vi "Digital (Pipelined Sample Clock) - Continuous Output.vi"() -> ()   [LabVIEW 2022 SP3]
doc: "This example demonstrates how to interface the NI 6536/7 to a synchronous DAC with an output enabled signal."
uses:
  <vilib>/Utility/error.llb/DialogType.ctl
  <vilib>/DAQmx/write.llb/DAQmx Write (Digital 1D Wfm NChan NSamp).vi
  <vilib>/DAQmx/create/channels.llb/DAQmx Create Channel (DO-Digital Output).vi
  <vilib>/DAQmx/configure/timing.llb/DAQmx Timing (Pipelined Sample Clock).vi
  <vilib>/Waveform/DWDTOps.llb/Digital Pattern Generator (Ramp).vi
  <vilib>/Waveform/DWDTOps.llb/DWDT Uncompress Digital.vi
  <vilib>/DAQmx/miscellaneous.llb/DAQmx Fill In Error Info.vi
  <resource>/objmgr/daqmx.rc
panel:
  in  "Pause Trigger Polarity":i32(ring)=10192 items=["High"=10192, "Low"=10214]
  in  "Data Active Level":i32(ring)=10095 items=["Active High"=10095, "Active Low"=10096]
  in  "Sample Clock Polarity":i32(ring)=10095 items=["Active High"=10095, "Active Low"=10096]
  in  "Handshaking?":bool
  in  "Pause Trigger Source Terminal":tag="/Dev1/PFI1" caption="Pause Trigger \nSource"
  in  "Data Active Output Terminal":tag="/Dev1/PFI0" caption="Data Active Output"
  in  "Sample Clock Output":tag="/Dev1/PFI1"
  in  "Samples per Channel per write":u32=1000 caption="Samples per Buffer"
  in  "Stop":bool
  out "Digital Waveform Graph":digitalwaveform[](graph)
  in  "Sample Rate":dbl=1000.0
  in  "Line(s)":tag="Dev1/port0/line0:7"
  # "Channel Settings"
  # "Generated Data"
  # "Timing Settings"
  # "Advanced Settings"
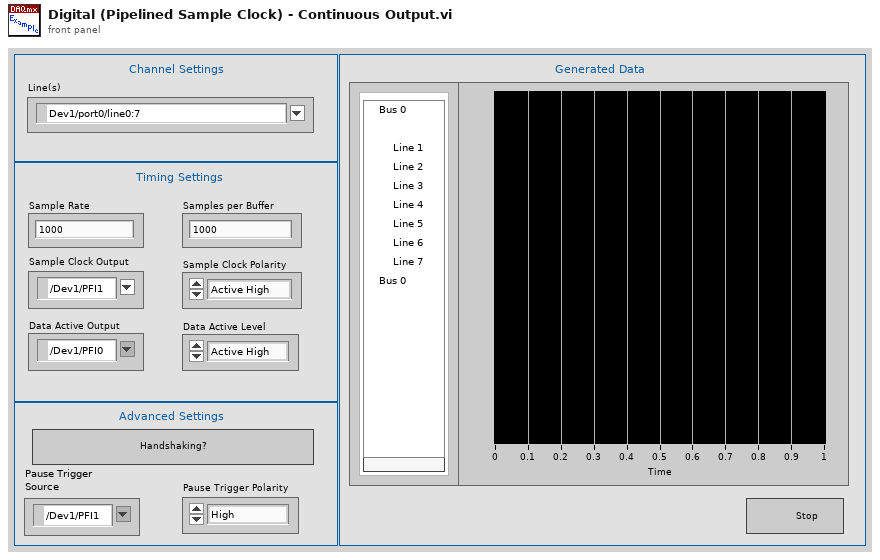
[diagram p1: front panel]
types:
  T1 = typedef "DialogType.ctl" = u16
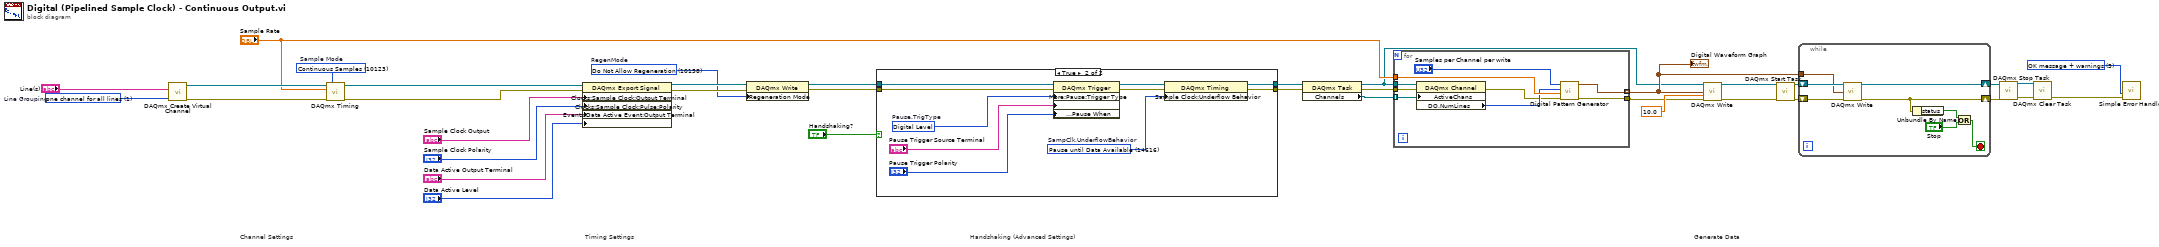
[diagram p0: block diagram]
diagram:
  w22 = T1 3 items=["no dialog", "OK message", "continue or stop message", "OK message + warnings", "continue/stop + warnings"] ("type of dialog (OK msg:1)")
  w10 = 10158 items=["Allow Regeneration"=10097, "Do Not Allow Regeneration"=10158]  # RegenMode
  w34 = 10123 items=["Finite Samples"=10178, "Continuous Samples"=10123, "Hardware Timed Single Point"=12522]  # Sample Mode
  w36 = 1 items=["one channel for each line", "one channel for all lines"]  # Line Grouping
  # "Timing Settings"
  # "Generate Data"
  # "Handshaking (Advanced Settings)"
  # "Channel Settings"
  n1 = call-poly <vilib>:"DAQmx Create Virtual Channel.vi"("lines"="Line(s)", "line grouping"=w36) -> ("task out"=w35:refnum<k21>, "error out"=w33:errorcluster)  [unwired: 12 in]
  n2 = call-poly <vilib>:"DAQmx Timing.vi"("task/channels in"=w35, "sample mode"=w34, "rate"="Sample Rate", "error in"=w33) -> ("task out"=w31:refnum<k21>, "error out"=w30:errorcluster)  [unwired: 10 in]
  n3 = property class="DAQmx Export Signal"(reference=w31, error in=w30, "Clocks:Sample Clock:Output Terminal"="Sample Clock Output", "Clocks:Sample Clock:Pulse:Polarity"="Sample Clock Polarity", "Events:Data Active Event:Output Terminal"="Data Active Output Terminal", "Events:Data Active Event:Level:Active Level"="Data Active Level") -> (reference out=w29:refnum<k21>, error out=w28:errorcluster)
  n4 = property class="DAQmx Write"(reference=w29, error in=w28, "Regeneration Mode"=w10) -> (reference out=w20:refnum<k21>, error out=w19:errorcluster)
  n5 = case shown="True" "Handshaking?" {
    tunnel: w20 -> [w38 w42]
    tunnel: w19 -> [w37 w45]
    tunnel: [w37 w43] -> w16
    tunnel: [w38 w40] -> w17
    frame False {
    }
    frame True {
      w46 = 14616 items=["Halt Output and Error"=14615, "Pause until Data Available"=14616]  # SampClk.UnderflowBehavior
      w48 = 10152 items=["Analog Level"=10101, "Analog Window"=10103, "Digital Level"=10152, "Digital Pattern"=10398, "None"=10230]  # Pause.TrigType
      n6 = property class="DAQmx Trigger"(reference=w42, error in=w45, "More:Pause:Trigger Type"=w48, "More:Pause:Digital Level:Source"="Pause Trigger Source Terminal", "More:Pause:Digital Level:Pause When"="Pause Trigger Polarity") -> (reference out=w41:refnum<k21>, error out=w44:errorcluster)
      n7 = property class="DAQmx Timing"(reference=w41, error in=w44, "Sample Clock:Underflow Behavior"=w46) -> (reference out=w40:refnum<k21>, error out=w43:errorcluster)
    }
  }
  n8 = property class="DAQmx Task"(reference=w17, error in=w16) -> (reference out=w6:refnum<k21>, error out=w15:errorcluster, "Channels"=w5:refnum<k21>[])
  n9 = for {
    tunnel: "Sample Rate" -> [w56]
    tunnel: [w55] -> w9 mode=indexing
    tunnel: [w54] -> w18
    tunnel: w15 -> [w50]
    tunnel: w6 -> [w53]
    tunnel: w5 -> [w52] mode=indexing
    n10 = property class="DAQmx Channel"(reference=w53, error in=w50, "ActiveChans"=w52) -> (error out=w49:errorcluster, "DO.NumLines"=w51:u32)  [unwired: 1 out]
    n11 = call-poly <vilib>:"Digital Pattern Generator.vi"("error in (no error)"=w49, "sample rate"=w56, "number of signals"=w51, "number of samples"="Samples per Channel per write") -> ("error out"=w54:errorcluster, "digital waveform"=w55:digitalwaveform)  [unwired: 6 in]
  }
  "Digital Waveform Graph" <- w9
  n12 = call-poly <vilib>:"DAQmx Write.vi"("task/channels in"=w6, "data"=w9, "timeout"=10.0 ("Write Timeout"), "error in"=w18) -> ("task out"=w24:refnum<k21>, "error out"=w25:errorcluster)  [unwired: 9 in, 1 out]
  n13 = call <vilib>:"DAQmx Start Task.vi"("task/channels in"=w24, "error in"=w25) -> ("task out"=w26:refnum<k21>, "error out"=w27:errorcluster)  [unwired: 12 in]
  n14 = while {
    shift-right: [w63] -> w4
    shift-left: w26 -> [w65]
    shift-right: [w62] -> w3
    shift-left: w27 -> [w64]
    tunnel: w9 -> [w59]
    stop <- w60 stop-if-true
    n15 = call-poly <vilib>:"DAQmx Write.vi"("task/channels in"=w65, "data"=w59, "error in"=w64) -> ("task out"=w63:refnum<k21>, "error out"=w62:errorcluster)  [unwired: 10 in, 1 out]
    n16 = Unbundle By Name(w62) -> ("status"=w61:bool)
    n17 = Or(x=w61, y="Stop") -> (x .or. y?=w60:bool)
  }
  n18 = call <vilib>:"DAQmx Stop Task.vi"("task/channels in"=w4, "error in"=w3) -> ("task out"=w2:refnum<k21>, "error out"=w1:errorcluster)  [unwired: 12 in]
  n19 = call <vilib>:"DAQmx Clear Task.vi"("task in"=w2, "error in"=w1) -> ("error out"=w21:errorcluster)  [unwired: 13 in]
  n20 = call <vilib>:"Simple Error Handler.vi"("type of dialog (OK msg:1)"=w22, "error in (no error)"=w21) -> ()  [unwired: 3 in, 5 out]
